vi "Import From Config.vi"(7 "selected path":path, 8 "error in":errorcluster, 9 "Overwrite Existing Channels?":bool=TRUE, 10 "Overwrite Device Settings?":bool=TRUE, 11 "Device Ref in":T1 format="%.0x") -> (0 "error out":errorcluster)   [LabVIEW 2020, in "Modbus Master System Explorer.lvlib"]
uses:
  Modbus Master System Explorer.lvlib
  <vilib>/NI VeriStand/Custom Device API/Custom Device Item Ref.ctl
  Modbus Type.ctl
  Shared/Controls/Data Model/Mapping.ctl
  Shared/Controls/Data Model/DataType.ctl
  <vilib>/NI VeriStand/Custom Device API/Custom Device Channel Type.ctl
  Shared/Constants.vi
  <vilib>/NI VeriStand/Custom Device Tools/Custom Device Utility Library/NI VeriStand - Search for Item by GUID.vi
  <vilib>/Utility/config.llb/Read Key (String).vi
  <vilib>/Utility/config.llb/Read Key (U32).vi
  <vilib>/NI VeriStand/Custom Device Tools/Custom Device Utility Library/NI VeriStand - Search for Item by Name.vi
  <vilib>/Utility/config.llb/NI_LVConfig.lvlib
  Shared/Modbus Master Shared.lvlib
  <vilib>/NI VeriStand/Custom Device Tools/Custom Device Utility Library/Custom Device Utility Library.lvlib
  <vilib>/NI VeriStand/Custom Device API/Custom Device API.lvlib
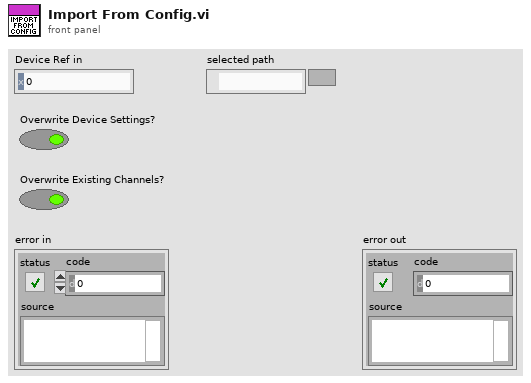
[diagram p1: front panel]
types:
  T1 = typedef "Custom Device API.lvlib/Custom Device Item Ref.ctl" = u64
  T2 = typedef "Custom Device API.lvlib/Custom Device Channel Type.ctl" = enum16{"Input", "Output"}
  T3 = typedef "Modbus Master Shared.lvlib/Mapping.ctl" = cluster{"DataType":T4, "Starting Address":u16, "Sub-Index (Bool)":u16, "VS Reference":T1}
  T4 = typedef "Modbus Master Shared.lvlib/DataType.ctl" = enum16{"Double", "Single", "I64", "I32", "I16", "I8", "U64", "U32", "U16", "U8", "Boolean"}
  T5 = typedef "NI_LVConfig.lvlib/Config Data RefNum.ctl" = refnum<k1>
  T6 = typedef "Modbus Master Shared.lvlib/Modbus Type.ctl" = enum16{"Coil", "Discrete Input", "Holding Register", "Input Register"}
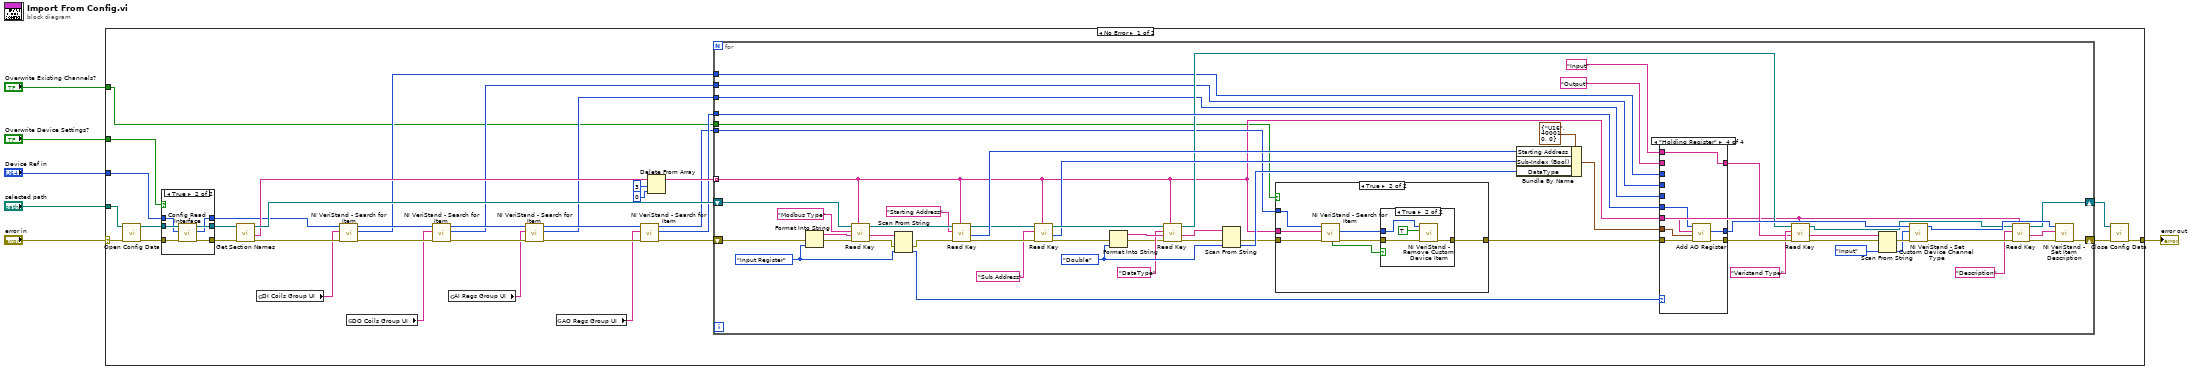
[diagram p0: block diagram]
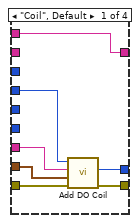
[diagram p5: hidden frame]
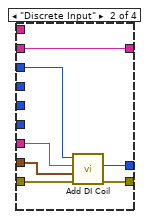
[diagram p6: hidden frame]
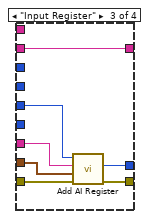
[diagram p7: hidden frame]
diagram:
  n1 = case shown="No Error" "error in" {
    selector: "error in" -> [w31 w148]
    tunnel: "selected path" -> [w41 _]
    tunnel: [w40 w148] -> w5
    tunnel: "Device Ref in" -> [w38 _]
    tunnel: "Overwrite Device Settings?" -> [w9 _]
    tunnel: "Overwrite Existing Channels?" -> [w7 _]
    frame No Error {
      n2 = call <vilib>:"Open Config Data.vi"("error in (no error)"=w31, "configuration file path"=w41) -> ("error out"=w30:errorcluster, "refnum"=w39:T5)  [unwired: 7 in, 1 out]
      n3 = case shown="True" w9 {
        tunnel: w39 -> [w42 w50]
        tunnel: w38 -> [w44 w49]
        tunnel: [w42 w48] -> w37
        tunnel: w30 -> [w43 w47]
        tunnel: [w43 w46] -> w29
        tunnel: [w44 w45] -> w15
        frame False {
        }
        frame True {
          n4 = call "Config Read Interface.vi"("error in (no error)"=w47, "Device Ref in"=w49, "Refnum in"=w50) -> ("error out"=w46:errorcluster, "Device Ref out"=w45:T1, "Refnum out"=w48:T5)  [unwired: 6 in]
        }
      }
      n5 = call <vilib>:"Get Section Names.vi"("error in (no error)"=w29, "refnum"=w37) -> ("error out"=w17:errorcluster, "section names"=w32:string[], "refnum out"=w34:T5)  [unwired: 7 in]
      n6 = global read "Constants.vi" "DI Coils Group UI"() -> (w14:string)
      n7 = call-poly <vilib>:"NI VeriStand - Search for Item.vi"("error in"=w17, "Item GUID"=w14, "Section Ref in"=w15) -> ("error out"=w22:errorcluster, "Item Ref"=w12:T1, "Section Ref out"=w21:T1)  [unwired: 5 in, 1 out]
      n8 = global read "Constants.vi" "DO Coils Group UI"() -> (w20:string)
      n9 = call-poly <vilib>:"NI VeriStand - Search for Item.vi"("error in"=w22, "Item GUID"=w20, "Section Ref in"=w21) -> ("error out"=w25:errorcluster, "Item Ref"=w13:T1, "Section Ref out"=w23:T1)  [unwired: 5 in, 1 out]
      n10 = global read "Constants.vi" "AI Regs Group UI"() -> (w19:string)
      n11 = call-poly <vilib>:"NI VeriStand - Search for Item.vi"("error in"=w25, "Item GUID"=w19, "Section Ref in"=w23) -> ("error out"=w26:errorcluster, "Item Ref"=w10:T1, "Section Ref out"=w24:T1)  [unwired: 5 in, 1 out]
      n12 = global read "Constants.vi" "AO Regs Group UI"() -> (w18:string)
      n13 = call-poly <vilib>:"NI VeriStand - Search for Item.vi"("error in"=w26, "Item GUID"=w18, "Section Ref in"=w24) -> ("error out"=w16:errorcluster, "Item Ref"=w11:T1, "Section Ref out"=w8:T1)  [unwired: 5 in, 1 out]
      n14 = Delete From Array(array=w32, length=3, index=0) -> (array with subset deleted=w33:string[])  [unwired: 1 out]
      n15 = for {
        tunnel: w33 -> [w56] mode=indexing
        shift-right: [w64] -> w27
        shift-left: w16 -> [w71]
        shift-right: [w60] -> w28
        shift-left: w34 -> [w72]
        tunnel: w13 -> [w82]
        tunnel: w12 -> [w83]
        tunnel: w11 -> [w104]
        tunnel: w10 -> [w81]
        tunnel: w8 -> [w57]
        tunnel: w7 -> [w55]
        w74 = DataType."Double" ("DataType")
        w76 = Modbus_Type."Input Register" ("Type")
        n16 = Format Into String(error in=w71, w76) -> (resulting string=w75:string, error out=w70:errorcluster)  [unwired: 2 in]
        n17 = call-poly <vilib>:"Read Key.vi"("section"=w56, "error in (no error)"=w70, "default value"=w75, "key"="Modbus Type", "refnum"=w72) -> ("error out"=w106:errorcluster, "value"=w105:string, "refnum out"=w103:T5)  [unwired: 3 in, 1 out]
        n18 = Scan From String(input string=w105, error in=w106, default 1=w76) -> (error out=w102:errorcluster, output 1=w84:T6)  [unwired: 2 in, 2 out]
        n19 = call-poly <vilib>:"Read Key.vi"("section"=w56, "error in (no error)"=w102, "key"="Starting Address", "refnum"=w103) -> ("error out"=w96:errorcluster, "value"=w100:u32, "refnum out"=w98:T5)  [unwired: 4 in, 1 out]
        n20 = call-poly <vilib>:"Read Key.vi"("section"=w56, "error in (no error)"=w96, "key"="Sub Address", "refnum"=w98) -> ("error out"=w52:errorcluster, "value"=w95:u32, "refnum out"=w97:T5)  [unwired: 4 in, 1 out]
        n21 = Format Into String(error in=w52, w74) -> (resulting string=w73:string, error out=w51:errorcluster)  [unwired: 2 in]
        n22 = call-poly <vilib>:"Read Key.vi"("section"=w56, "error in (no error)"=w51, "default value"=w73, "key"="DataType", "refnum"=w97) -> ("error out"=w93:errorcluster, "value"=w94:string, "refnum out"=w88:T5)  [unwired: 3 in, 1 out]
        n23 = Scan From String(input string=w94, error in=w93, default 1=w74) -> (error out=w54:errorcluster, output 1=w92:T4)  [unwired: 2 in, 2 out]
        n24 = case shown="True" w55 {
          tunnel: w57 -> [_ w114]
          tunnel: w56 -> [_ w113]
          tunnel: w54 -> [w107 w109]
          tunnel: [w107 w108] -> w53
          frame False {
          }
          frame True {
            n25 = call-poly <vilib>:"NI VeriStand - Search for Item.vi"("error in"=w109, "Item Name"=w113, "Section Ref in"=w114) -> ("error out"=w110:errorcluster, "Item Ref"=w111:T1, "Found"=w112:bool)  [unwired: 5 in, 1 out]
            n26 = case shown="True" w112 {
              tunnel: w111 -> [_ w119]
              tunnel: w110 -> [w115 w118]
              tunnel: [w115 w117] -> w108
              frame False {
              }
              frame True {
                n27 = call <vilib>:"NI VeriStand - Remove Custom Device Item.vi"("error in (no error)"=w118, "Force Delete (F)"=TRUE, "Item Ref in"=w119) -> ("error out"=w117:errorcluster)  [unwired: 7 in, 1 out]
              }
            }
          }
        }
        n28 = Bundle By Name(cluster=T3 {"DataType"=enum."U16", "Starting Address"=40001, "Sub-Index (Bool)"=0, "VS Reference"=0} ("Mapping"), "Starting Address"=w100, "Sub-Index (Bool)"=w95, "DataType"=w92) -> (w99:T3)
        n29 = case shown="\"Holding Register\"" w84 {
          tunnel: w104 -> [_ _ _ w147]
          tunnel: w56 -> [w123 w129 w135 w146]
          tunnel: w99 -> [w124 w130 w140 w145]
          tunnel: w53 -> [w126 w133 w134 w144]
          tunnel: [w122 w131 w138 w143] -> w91
          tunnel: [w125 w132 w139 w142] -> w90
          tunnel: w83 -> [_ w128 _ _]
          tunnel: w82 -> [w121 _ _ _]
          tunnel: w81 -> [_ _ w136 _]
          tunnel: [w120 w127 w137 w141] -> w79
          tunnel: "Input" ("default value") -> [w120 _ _ w141]
          tunnel: "Output" ("default value") -> [_ w127 w137 _]
          frame "Coil", Default {
            n30 = call "Add DO Coil.vi"("error in (no error)"=w126, "Mapping"=w124, "Label"=w123, "Node Ref In"=w121) -> ("error out"=w125:errorcluster, "Channel Ref"=w122:T1)  [unwired: 5 in, 1 out]
          }
          frame "Discrete Input" {
            n31 = call "Add DI Coil.vi"("error in (no error)"=w133, "Mapping"=w130, "Label"=w129, "Node Ref In"=w128) -> ("error out"=w132:errorcluster, "Channel Ref Out"=w131:T1)  [unwired: 5 in, 1 out]
          }
          frame "Input Register" {
            n32 = call "Add AI Register.vi"("error in (no error)"=w134, "Mapping"=w140, "Label"=w135, "Node Ref In"=w136) -> ("error out"=w139:errorcluster, "Channel Ref out"=w138:T1)  [unwired: 5 in, 1 out]
          }
          frame "Holding Register" {
            n33 = call "Add AO Register.vi"("error in (no error)"=w144, "Mapping"=w145, "Label"=w146, "Node Ref In"=w147) -> ("error out"=w142:errorcluster, "Channel Ref out"=w143:T1)  [unwired: 5 in, 1 out]
          }
        }
        n34 = call-poly <vilib>:"Read Key.vi"("section"=w56, "error in (no error)"=w90, "default value"=w79, "key"="Veristand Type", "refnum"=w88) -> ("error out"=w89:errorcluster, "value"=w86:string, "refnum out"=w61:T5)  [unwired: 3 in, 1 out]
        n35 = Scan From String(input string=w86, default 1=Custom_Device_Channel_Type."Input" ("Type")) -> (output 1=w85:T2)  [unwired: 3 in, 3 out]
        n36 = call <vilib>:"NI VeriStand - Set Custom Device Channel Type.vi"("error in (no error)"=w89, "Type"=w85, "Channel Ref in"=w91) -> ("error out"=w63:errorcluster, "Channel Ref out"=w65:T1)  [unwired: 7 in]
        n37 = call-poly <vilib>:"Read Key.vi"("section"=w56, "error in (no error)"=w63, "key"="Description", "refnum"=w61) -> ("error out"=w62:errorcluster, "value"=w58:string, "refnum out"=w60:T5)  [unwired: 4 in, 1 out]
        n38 = call <vilib>:"NI VeriStand - Set Item Description.vi"("error in (no error)"=w62, "Description"=w58, "Item Ref in"=w65) -> ("error out"=w64:errorcluster)  [unwired: 6 in, 2 out]
      }
      n39 = call <vilib>:"Close Config Data.vi"("error in (no error)"=w27, "refnum"=w28) -> ("error out"=w40:errorcluster)  [unwired: 8 in, 1 out]
    }
    frame Error {
    }
  }
  "error out" <- w5
